vi "Read Process.vi"(8 "error in (no error)":errorcluster, 11 "Debug Data In":refnum<class "Debug Data.lvclass">) -> (0 "error out":errorcluster, 2 "Process":string, 3 "Debug Data Out":refnum<class "Debug Data.lvclass">)   [LabVIEW 2020, in "Debug Data.lvclass"]
uses:
  Debug Data.lvclass
  Debug Data.lvclass/Debug Data.ctl
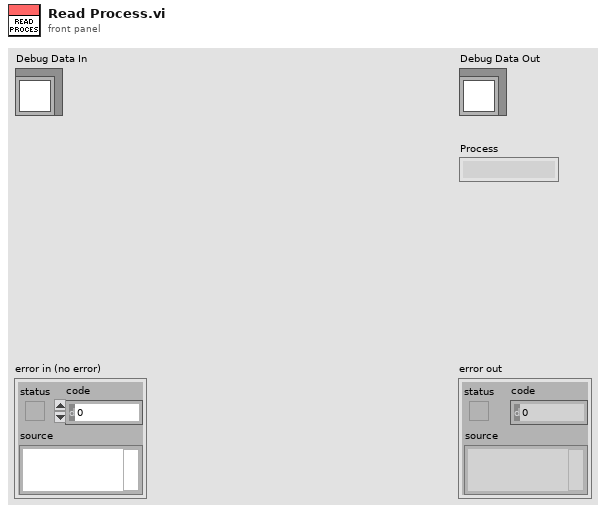
[diagram p1: front panel]
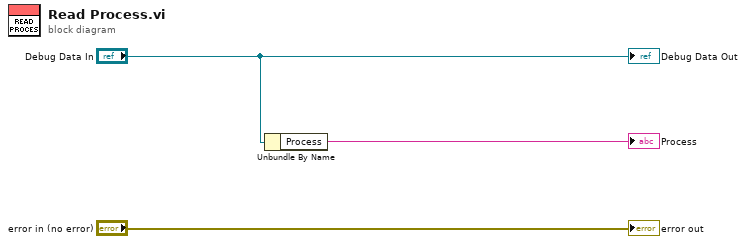
[diagram p0: block diagram]
diagram:
  n1 = Unbundle By Name("Debug Data In") -> ("Process"=→"Process":string)
  "error out" <- "error in (no error)"
  "Debug Data Out" <- "Debug Data In"
